vi "Random Number (Range).vi"   [LabVIEW 2020]
doc: "Generates a random value from a specified range. Wire data to the <B>upper bound</B> or <B>lower bound</B> input to determine the polymorphic instance to use or manually select the instance."
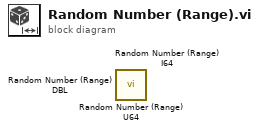
[diagram p0: block diagram]
diagram:
  n1 = call <vilib>:"Random Number (Range) U64.vi"() -> ()  [unwired: 11 in, 1 out]
  n2 = call <vilib>:"Random Number (Range) I64.vi"() -> ()  [unwired: 11 in, 1 out]
  n3 = call <vilib>:"Random Number (Range) DBL.vi"() -> ()  [unwired: 11 in, 1 out]
